vi "ConvertInsightPropertyToTdmsProperty_ChannelId.vi"(8 "Insight Channels":T1[](array[typedef]), 9 "Tdms Property Name":string, 10 "Insight Property Name":string, 11 "Insight Properties":T2[](array[typedef])) -> (3 "Tdms Properties":T4[](array[typedef]))   [LabVIEW 2017, in "Tdms.lvlib"]
uses:
  <vilib>/addons/InsightCM/Utilities/Tdms/Tdms.lvlib
  <vilib>/addons/InsightCM/MessageBus/Base/controls/KeyValuePair.ctl
  <vilib>/addons/InsightCM/Utilities/Tdms/controls/Property.ctl
  <vilib>/addons/InsightCM/MessageBus/Base/controls/R2_Channel.ctl
  <vilib>/addons/InsightCM/MessageBus/Base/controls/Metric.ctl
  <vilib>/addons/InsightCM/Utilities/PropertyHelpers/PropertyHelpers.lvlib
  <vilib>/addons/InsightCM/Utilities/DeviceModelHelpers/DeviceModelHelpers.lvlib
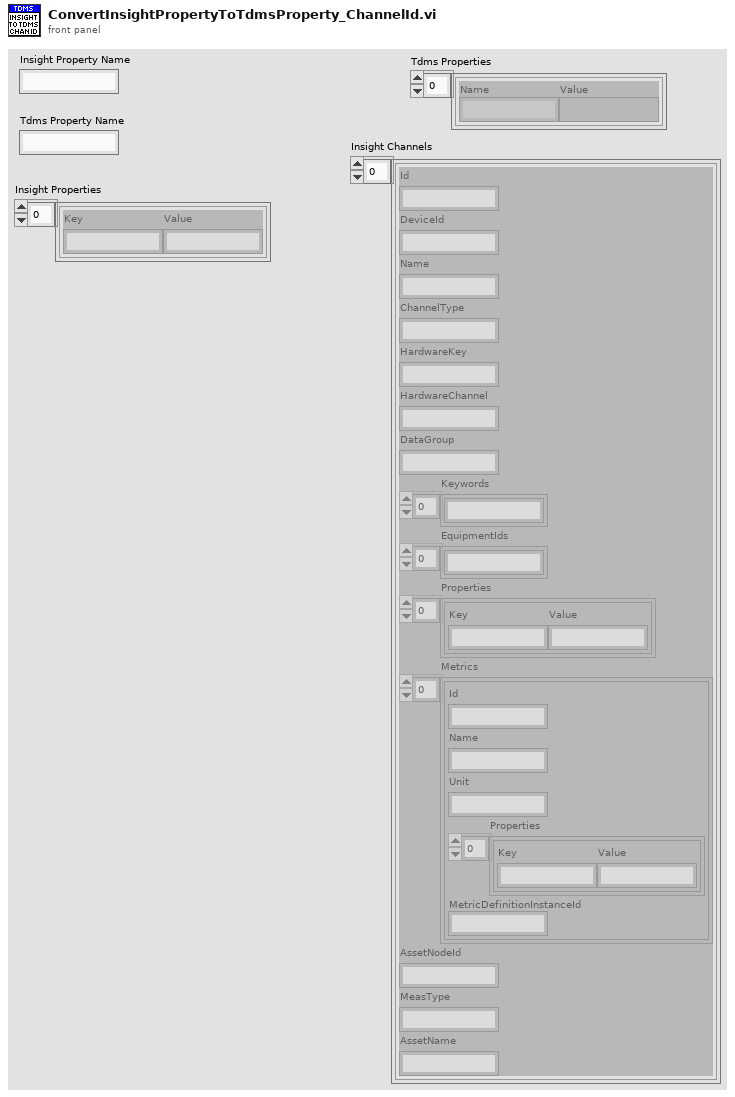
[diagram p1: front panel]
types:
  T1 = typedef "R2_Channel.ctl" = cluster{"Id":string, "DeviceId":string, "Name":string, "ChannelType":string, "HardwareKey":string, "HardwareChannel":string, "DataGroup":string, "Keywords":string[], "EquipmentIds":string[], "Properties":T2[], "Metrics":T3[], "AssetNodeId":string, "MeasType":string, "AssetName":string}
  T2 = typedef "KeyValuePair.ctl" = cluster{"Key":string, "Value":string}
  T3 = typedef "Metric.ctl" = cluster{"Id":string, "Name":string, "Unit":string, "Properties":T2[], "MetricDefinitionInstanceId":string}
  T4 = typedef "Tdms.lvlib/Property.ctl" = cluster{"Name":string, "Value":variant}
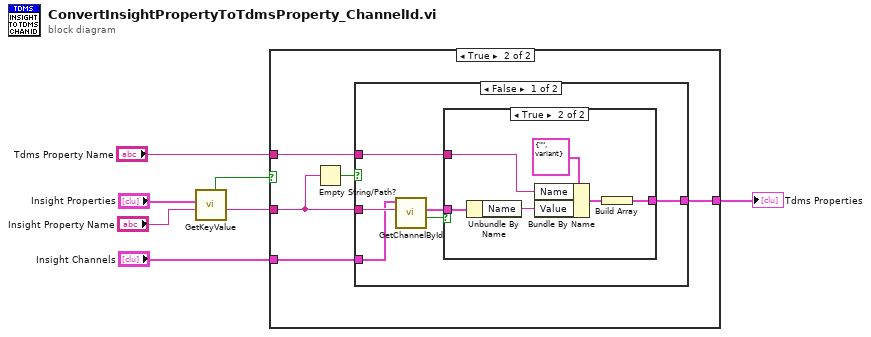
[diagram p0: block diagram]
diagram:
  n1 = call <vilib>:"GetKeyValue.vi"("key"="Insight Property Name", "key value pairs"="Insight Properties") -> ("value"=w2:string, "found"=w5:bool)  [unwired: 7 in, 1 out]
  n2 = case shown="True" w5 {
    tunnel: "Tdms Property Name" -> [_ w12]
    tunnel: w2 -> [_ w10]
    tunnel: [_ w11] -> w6
    tunnel: "Insight Channels" -> [_ w8]
    frame False {
    }
    frame True {
      n3 = Empty String/Path?(string/path=w10) -> (empty?=w9:bool)
      n4 = case shown="False" w9 {
        tunnel: w12 -> [w16 _]
        tunnel: w10 -> [w17 _]
        tunnel: [w18 _] -> w11
        tunnel: w8 -> [w13 _]
        frame False {
          n5 = call <vilib>:"GetChannelById.vi"("channel id"=w17, "channels in"=w13) -> ("found"=w15:bool, "channel"=w14:T1)  [unwired: 7 in, 1 out]
          n6 = case shown="True" w15 {
            tunnel: [_ w22] -> w18
            tunnel: w16 -> [_ w21]
            tunnel: w14 -> [_ w20]
            frame False {
            }
            frame True {
              n7 = Unbundle By Name(w20) -> ("Name"=w19:string)
              n8 = Bundle By Name(cluster=T4 {"Name"="", "Value"=variant} ("Property"), "Name"=w21, "Value"=w19) -> (w23:T4)
              n9 = Build Array(w23) -> (w22:T4[])
            }
          }
        }
        frame True {
        }
      }
    }
  }
  "Tdms Properties" <- w6
